vi "获取公式存入关键参数.vi"(8 "error in (no error)":errorcluster caption="错误输入（无错误）", 9 "量程":u16, 10 "flowid":u16, 11 "id":u16) -> (0 "error out":errorcluster caption="错误输出")   [LabVIEW 2016, in "斯坦道总氮.lvlib"]
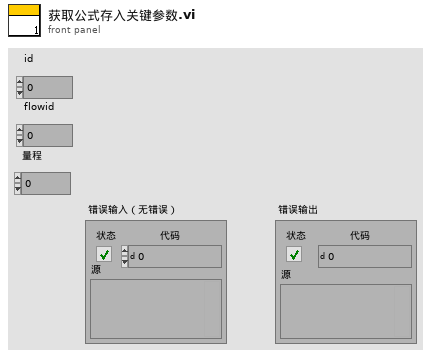
[diagram p1: front panel]
types:
  T1 = typedef "斯坦道总氮.lvlib/关键参数.ctl" = cluster{"测量量程":sgl, "测量检出限":sgl, "测量精度":sgl, "测量间隔":sgl, "消解温度":sgl, "消解时长":sgl, "三项式系数":sgl, "二次多项式系数":sgl, "曲线斜率":sgl, "曲线截距":sgl, "线性相关系数":sgl, "空白校准时间":timestamp, "标样校准时间":timestamp, "测量信号值":sgl, "稀释倍数":sgl, "空白标定系数":sgl, "量程系数":sgl}
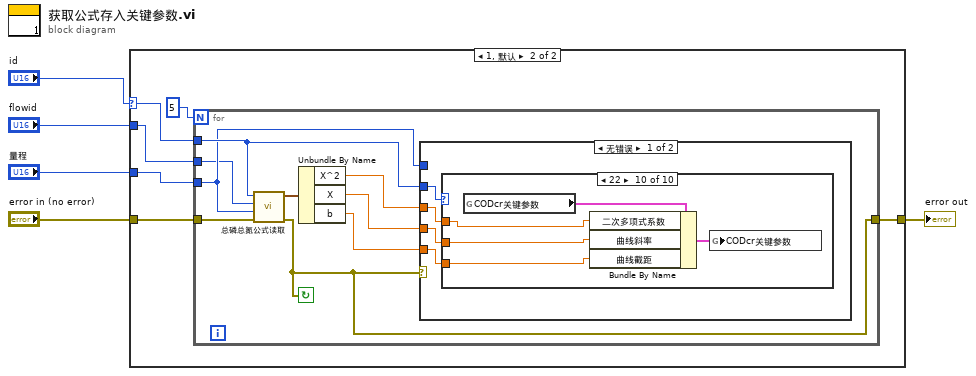
[diagram p0: block diagram]
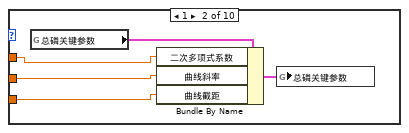
[diagram p4: hidden frame]
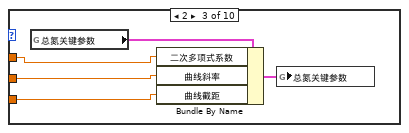
[diagram p5: hidden frame]
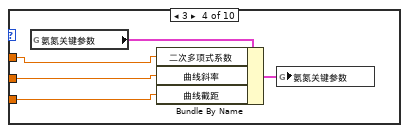
[diagram p6: hidden frame]
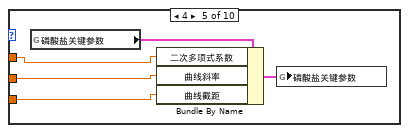
[diagram p7: hidden frame]
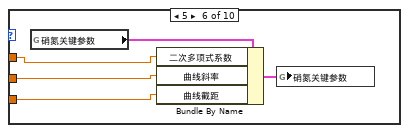
[diagram p8: hidden frame]
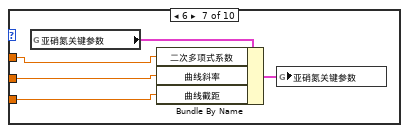
[diagram p9: hidden frame]
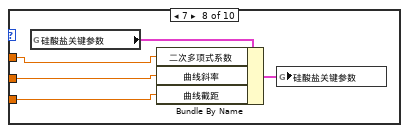
[diagram p10: hidden frame]
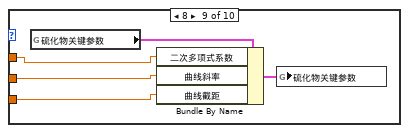
[diagram p11: hidden frame]
diagram:
  n1 = case shown="1, 默认" "id" {
    selector: "id" -> [_ w7]
    tunnel: "flowid" -> [_ w11]
    tunnel: "量程" -> [_ w10]
    tunnel: "error in (no error)" -> [w6 w9]
    tunnel: [w6 w8] -> w2
    frame 0 {
    }
    frame 1, Default {
      n2 = for {
        N: 5 -> [_]
        tunnel: w10 -> [w16]
        tunnel: w11 -> [w15]
        tunnel: w7 -> [w17]
        tunnel: w9 -> [w14]
        tunnel: [w13] -> w8
        stop <- w13 continue-if-true
        n3 = call "总磷总氮公式读取.vi"("error in (no error)"=w14, "量程"=w16, "测量模式"=w15, "测量参数"=w17) -> ("error out"=w13:errorcluster, "公式"=w21:cluster{"X^2":dbl, "X":dbl, "b":dbl})  [unwired: 6 in]
        n4 = Unbundle By Name(w21) -> ("X^2"=w20:dbl, "X"=w19:dbl, "b"=w18:dbl)
        n5 = case shown="无错误" w13 {
          tunnel: w20 -> [w25 _]
          tunnel: w19 -> [w24 _]
          tunnel: w18 -> [w23 _]
          tunnel: w17 -> [w22 _]
          tunnel: w16 -> [_ _]
          frame No Error {
            n6 = case shown="22" w22 {
              tunnel: w25 -> [_ w28 w33 w38 w43 w48 w53 w58 w63 w68]
              tunnel: w24 -> [_ w27 w32 w37 w42 w47 w52 w57 w62 w67]
              tunnel: w23 -> [_ w26 w31 w36 w41 w46 w51 w56 w61 w66]
              frame 0, Default {
              }
              frame 1 {
                n7 = global read "VAR总磷总氮全局变量.vi" "总磷关键参数"() -> (w29:T1)
                n8 = Bundle By Name(cluster=w29, "二次多项式系数"=w28, "曲线斜率"=w27, "曲线截距"=w26) -> (w30:T1)
                n9 = global write "VAR总磷总氮全局变量.vi" "总磷关键参数"(w30) -> ()
              }
              frame 2 {
                n10 = global read "VAR总磷总氮全局变量.vi" "总氮关键参数"() -> (w34:T1)
                n11 = Bundle By Name(cluster=w34, "二次多项式系数"=w33, "曲线斜率"=w32, "曲线截距"=w31) -> (w35:T1)
                n12 = global write "VAR总磷总氮全局变量.vi" "总氮关键参数"(w35) -> ()
              }
              frame 3 {
                n13 = global read "VAR总磷总氮全局变量.vi" "氨氮关键参数"() -> (w39:T1)
                n14 = Bundle By Name(cluster=w39, "二次多项式系数"=w38, "曲线斜率"=w37, "曲线截距"=w36) -> (w40:T1)
                n15 = global write "VAR总磷总氮全局变量.vi" "氨氮关键参数"(w40) -> ()
              }
              frame 4 {
                n16 = global read "VAR总磷总氮全局变量.vi" "磷酸盐关键参数"() -> (w44:T1)
                n17 = Bundle By Name(cluster=w44, "二次多项式系数"=w43, "曲线斜率"=w42, "曲线截距"=w41) -> (w45:T1)
                n18 = global write "VAR总磷总氮全局变量.vi" "磷酸盐关键参数"(w45) -> ()
              }
              frame 5 {
                n19 = global read "VAR总磷总氮全局变量.vi" "硝氮关键参数"() -> (w49:T1)
                n20 = Bundle By Name(cluster=w49, "二次多项式系数"=w48, "曲线斜率"=w47, "曲线截距"=w46) -> (w50:T1)
                n21 = global write "VAR总磷总氮全局变量.vi" "硝氮关键参数"(w50) -> ()
              }
              frame 6 {
                n22 = global read "VAR总磷总氮全局变量.vi" "亚硝氮关键参数"() -> (w54:T1)
                n23 = Bundle By Name(cluster=w54, "二次多项式系数"=w53, "曲线斜率"=w52, "曲线截距"=w51) -> (w55:T1)
                n24 = global write "VAR总磷总氮全局变量.vi" "亚硝氮关键参数"(w55) -> ()
              }
              frame 7 {
                n25 = global read "VAR总磷总氮全局变量.vi" "硅酸盐关键参数"() -> (w59:T1)
                n26 = Bundle By Name(cluster=w59, "二次多项式系数"=w58, "曲线斜率"=w57, "曲线截距"=w56) -> (w60:T1)
                n27 = global write "VAR总磷总氮全局变量.vi" "硅酸盐关键参数"(w60) -> ()
              }
              frame 8 {
                n28 = global read "VAR总磷总氮全局变量.vi" "硫化物关键参数"() -> (w64:T1)
                n29 = Bundle By Name(cluster=w64, "二次多项式系数"=w63, "曲线斜率"=w62, "曲线截距"=w61) -> (w65:T1)
                n30 = global write "VAR总磷总氮全局变量.vi" "硫化物关键参数"(w65) -> ()
              }
              frame 22 {
                n31 = global read "VAR总磷总氮全局变量.vi" "CODcr关键参数"() -> (w69:T1)
                n32 = Bundle By Name(cluster=w69, "二次多项式系数"=w68, "曲线斜率"=w67, "曲线截距"=w66) -> (w70:T1)
                n33 = global write "VAR总磷总氮全局变量.vi" "CODcr关键参数"(w70) -> ()
              }
            }
          }
          frame Error {
          }
        }
      }
    }
  }
  "error out" <- w2
